vi "Build Tool.vi"(6 "String":string, 7 "Ignored":string[](array[string])=["error in"], 8 "error in (no error)":errorcluster, 9 "Description":string, 11 "VI Refnum":refnum<vi>) -> (0 "error out":errorcluster, 3 "array":T1)   [LabVIEW 2025, in "MCP Server.lvlib"]
doc: "Creates a new Tool object from a VI."
uses:
  MCP Server.lvlib
  Tool Data.ctl
  Input Parameter.ctl
  Output Parameter.ctl
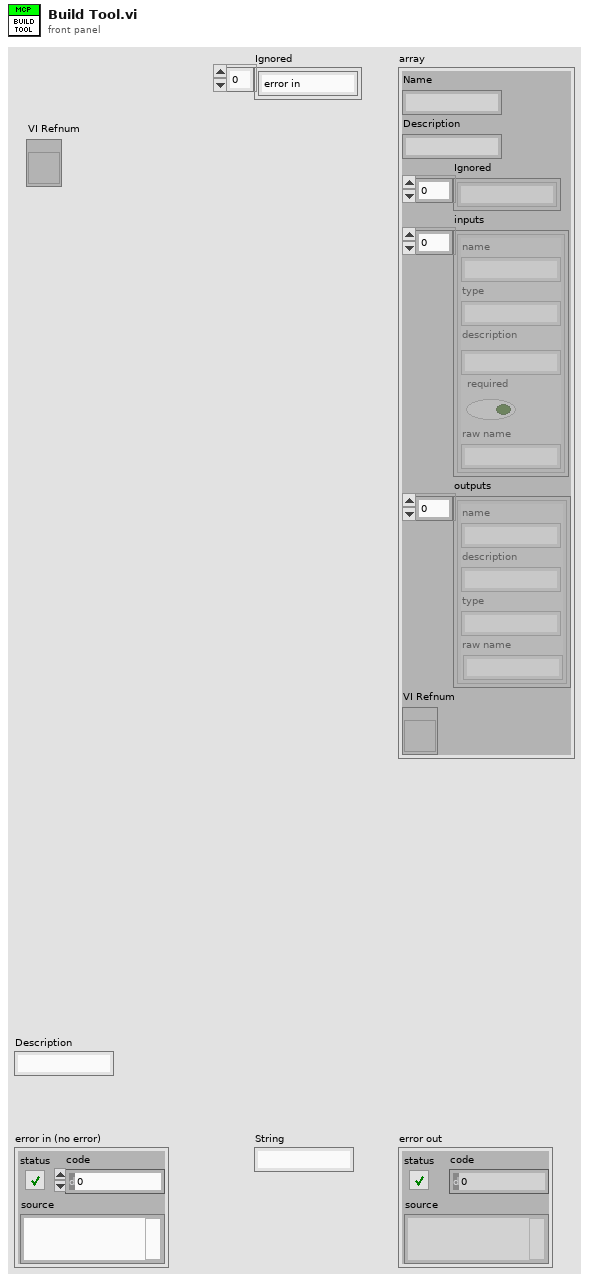
[diagram p1: front panel]
types:
  T1 = typedef "MCP Server.lvlib/Tool Data.ctl" = cluster{"Name":string, "Description":string, "Ignored":string[], "inputs":T2[], "outputs":T3[], "VI Refnum":refnum<vi>}
  T2 = typedef "MCP Server.lvlib/Input Parameter.ctl" = cluster{"name":string, "type":string, "description":string, "required":bool, "raw name":string}
  T3 = typedef "MCP Server.lvlib/Output Parameter.ctl" = cluster{"name":string, "description":string, "type":string, "raw name":string}
  T4 = typedef "MCP Server.lvlib/Terminal.ctl" = cluster{"Name":string, "Type":string, "IsIndicator?":bool, "IsRequired?":bool, "Description":string, "sub type":string, "array dimensions":i32}
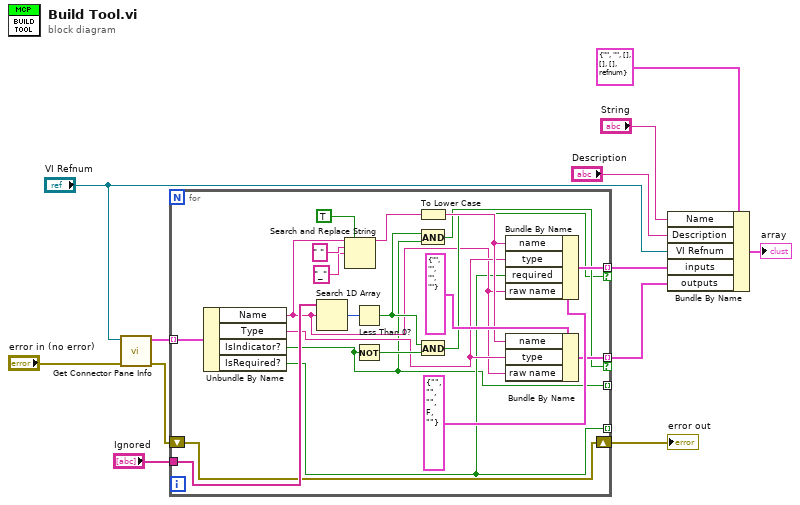
[diagram p0: block diagram]
diagram:
  n1 = call "Get Connector Pane Info.vi"("error in (no error)"="error in (no error)", "vi reference"="VI Refnum") -> ("error out"=w4:errorcluster, "Terminals"=w3:T4[])  [unwired: 8 in]
  n2 = for {
    tunnel: [w14] -> _ mode=indexing
    tunnel: [w32] -> w9 mode=indexing if=w27
    tunnel: [w29] -> w10 mode=indexing if=w28
    tunnel: "Ignored" -> [w25]
    shift-right: [w22] -> w11
    shift-left: w4 -> [w22]
    tunnel: [w13] -> _ mode=indexing
    tunnel: w3 -> [w17] mode=indexing
    n3 = Unbundle By Name(w17) -> ("Name"=w15:string, "Type"=w16:string, "IsIndicator?"=w13:bool, "IsRequired?"=w14:bool)
    n4 = Search 1D Array(1D array=w25, element=w15) -> (index of element=w24:i32)  [unwired: 1 in]
    n5 = Search and Replace String(replace all?=TRUE ("replace all? (F)"), input string=w15, search string=" ", replace string="_" ("replace string (\"\")")) -> (result string=w21:string)  [unwired: 4 in, 3 out]
    n6 = Less Than 0?(x=w24) -> (x < 0?=w23:bool)
    n7 = Not(x=w13) -> (.not. x?=w26:bool)
    n8 = To Lower Case(string=w21) -> (all lower case string=w30:string)
    n9 = And(x=w23, y=w13) -> (x .and. y?=w28:bool)
    n10 = And(x=w23, y=w26) -> (x .and. y?=w27:bool)
    n11 = Bundle By Name(cluster=T2 {"name"="", "type"="", "description"="", "required"=FALSE, "raw name"=""} ("Cluster"), "name"=w30, "type"=w16, "required"=w14, "raw name"=w15) -> (w32:T2)
    n12 = Bundle By Name(cluster=T3 {"name"="", "description"="", "type"="", "raw name"=""} ("outputs"), "name"=w30, "type"=w16, "raw name"=w15) -> (w29:T3)
  }
  "error out" <- w11
  n13 = Bundle By Name(cluster=T1 {"Name"="", "Description"="", "Ignored"=[], "inputs"=[], "outputs"=[], "VI Refnum"=refnum} ("Tool Data"), "Name"="String", "Description"="Description", "VI Refnum"="VI Refnum", "inputs"=w9, "outputs"=w10) -> (→"array":T1)
